vi "仪器电源管理.vi"() -> ()   [LabVIEW 2016, in "环境动力监测库.lvlib" / "电源管理库.lvlib"]
uses:
  <vilib>/Utility/miscctls.llb/LVPointTypeDef.ctl
panel:
  out "R115":i16 caption="灯带关闭时间"
  out "R114":i16 caption="灯带开启时间"
  in  "视频监控":bool
  in  "照明":bool
  in  "前门灯带":bool
  in  "侧边灯带":bool
  in  "电源控制":T1
  in  "副屏看门狗启用":u16(ring) caption="副屏看门狗启用：" items=["关闭", "打开"]
  in  "副屏看门狗设置":u16 caption="副屏看门狗设置："
  out "副屏看门狗计时":u16 caption="副屏看门狗计时："
  in  "主屏看门狗启用":u16(ring) caption="主屏看门狗启用：" items=["关闭", "打开"]
  in  "主屏看门狗设置":u16 caption="主屏看门狗设置："
  out "主屏看门狗计时":u16 caption="主屏看门狗计时："
  # "仪器电源管理"
  # "s"
  # "s"
  # "s"
  # "s"
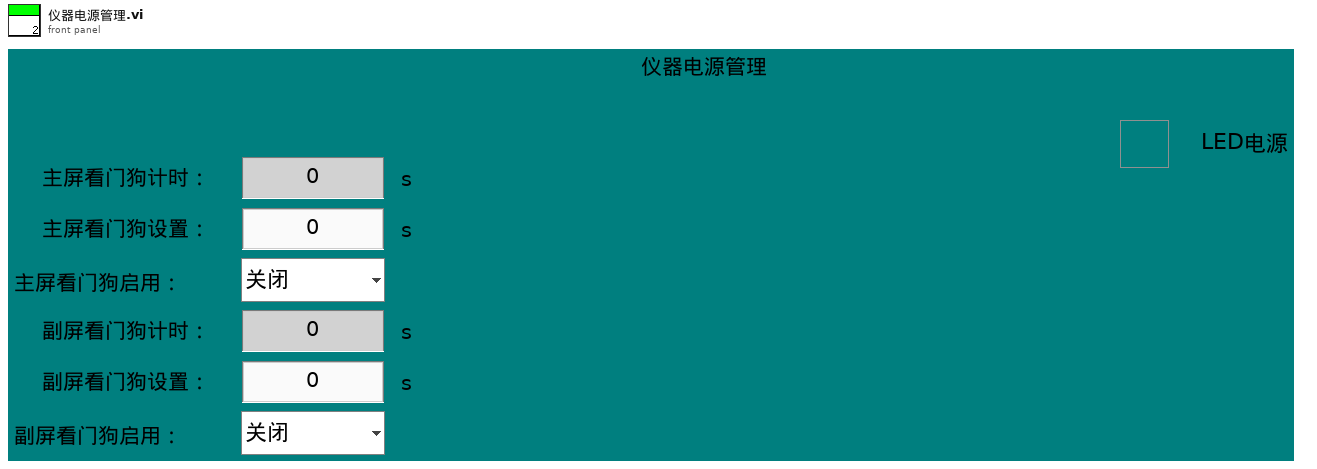
[diagram p1: front panel]
types:
  T1 = cluster{"氨氮电源":bool, "总磷电源":bool, "总氮电源":bool, "多参数电源":bool, "CODMn电源":bool, "CODCr电源":bool, "LED电源":bool}
  T2 = typedef "LVPointTypeDef.ctl" = cluster{"Horizontal":i16, "Vertical":i16}
  T3 = cluster{"采配水启用":bool, "CODMn启用":bool, "CODcr启用":bool, "氨氮启用":bool, "总磷启用":bool, "质控单元启用":bool, "流量计启用":bool, "电源管理启用":bool, "其他启用":bool, "多参数启用":bool, "超标留样启用":bool, "总氮启用":bool, "运行模式":enum16{"维护模式", "常规模式", "应急模式", "质控模式"}}
  T4 = cluster{"状态":cluster{"R0":i16, "R1":i16, "R2":i16, "R3":i16, "R4":i16, "R5":i16, "R6":i16, "R7":i16, "R8":i16, "R9":i16, "R10":i16, "R11":i16, "R12":i16, "R13":i16, "R14":i16, "R15":i16, "R16":i16, "R17":i16, "R18":i16, "R19":i16, "R20":i16, "R21":i16, "R22":i16, "R23":i16, "R24":i16, "R25":i16, "R26":i16, "R27":i16, "R28":i16, "R29":i16, "R30":i16, "R31":i16, "R32":i16, "R33":i16, "R34":i16, "R35":i16, "R36":i16, "R37":i16, "R38":i16, "R39":i16}, "输入状态":bool[], "输出状态":bool[], "参数设置":cluster{"R100":i16, "R101":i16, "R102":i16, "R103":i16, "R104":i16, "R105":i16, "R106":i16, "R107":i16, "R108":i16, "R109":i16, "R110":i16, "R111":i16, "R112":i16, "R113":i16, "R114":i16, "R115":i16, "R116":i16, "R117":i16, "R118":i16, "R119":i16, "R120":i16, "R121":i16, "R122":i16, "R123":i16}, "转换值":cluster{"AD0":sgl, "AD1":sgl, "AD2":sgl, "AD3":sgl, "AD4":sgl, "AD5":sgl}}
  T5 = cluster{"R100":i16, "R101":i16, "R102":i16, "R103":i16, "R104":i16, "R105":i16, "R106":i16, "R107":i16, "R108":i16, "R109":i16, "R110":i16, "R111":i16, "R112":i16, "R113":i16, "R114":i16, "R115":i16, "R116":i16, "R117":i16, "R118":i16, "R119":i16, "R120":i16, "R121":i16, "R122":i16, "R123":i16}
  T6 = cluster{"R0":i16, "R1":i16, "R2":i16, "R3":i16, "R4":i16, "R5":i16, "R6":i16, "R7":i16, "R8":i16, "R9":i16, "R10":i16, "R11":i16, "R12":i16, "R13":i16, "R14":i16, "R15":i16, "R16":i16, "R17":i16, "R18":i16, "R19":i16, "R20":i16, "R21":i16, "R22":i16, "R23":i16, "R24":i16, "R25":i16, "R26":i16, "R27":i16, "R28":i16, "R29":i16, "R30":i16, "R31":i16, "R32":i16, "R33":i16, "R34":i16, "R35":i16, "R36":i16, "R37":i16, "R38":i16, "R39":i16}
  T7 = cluster{"命令":string, "data":cluster{"starting address":u16, "coil values":bool[]}}
  T8 = cluster{"命令":string, "数据":cluster{"starting address":u16, "holding register values":u16[]}}
  T9 = cluster{"命令":string, "数据":cluster{"starting address":u16, "holding register value":u16}}
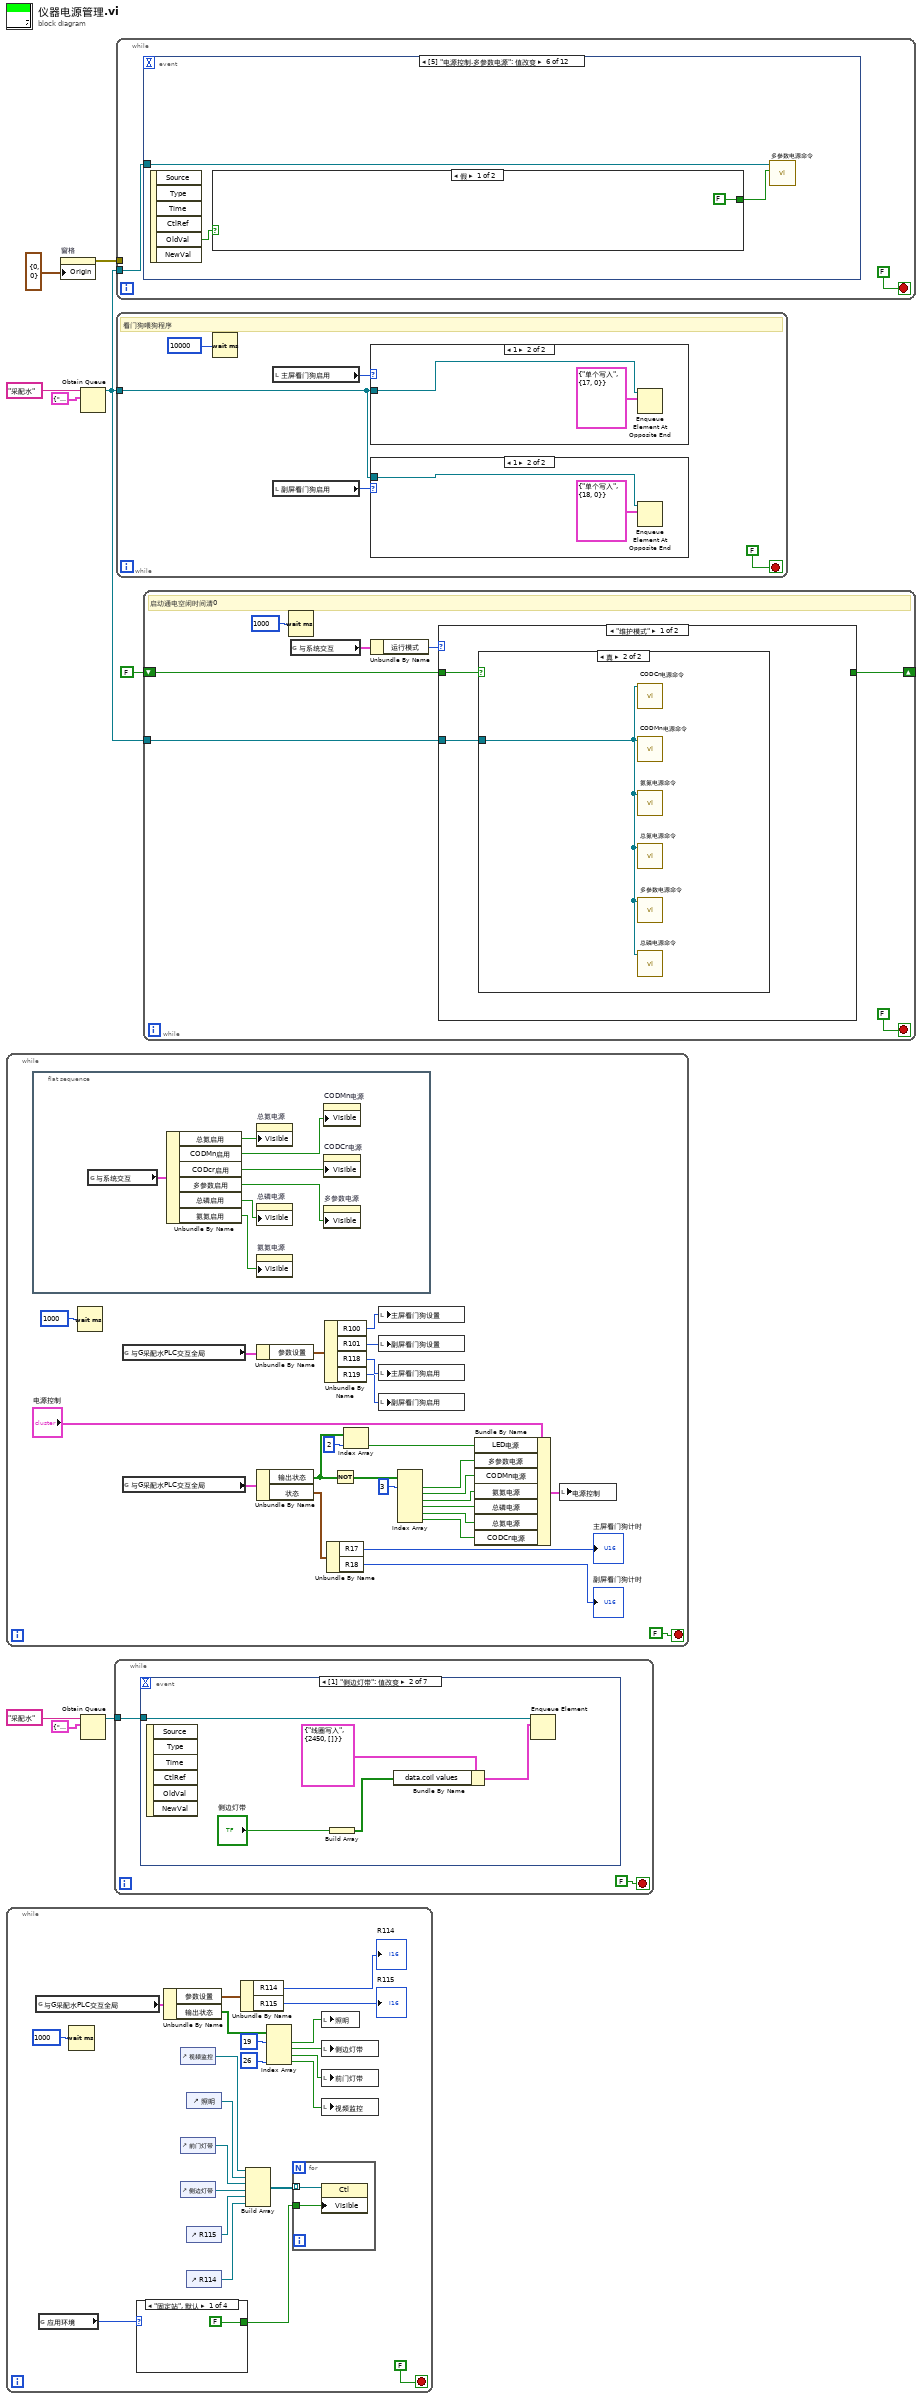
[diagram p0: block diagram]
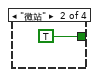
[diagram p2: hidden frame]
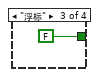
[diagram p3: hidden frame]
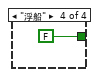
[diagram p4: hidden frame]
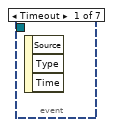
[diagram p5: hidden frame]
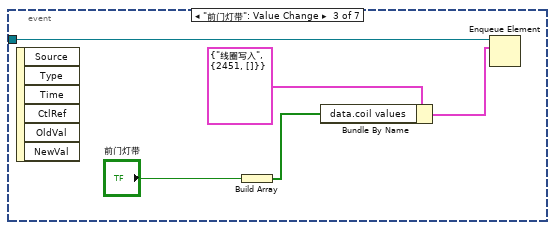
[diagram p6: hidden frame]
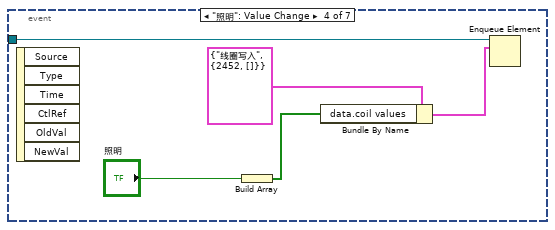
[diagram p7: hidden frame]
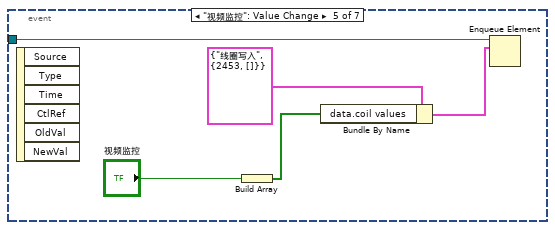
[diagram p8: hidden frame]
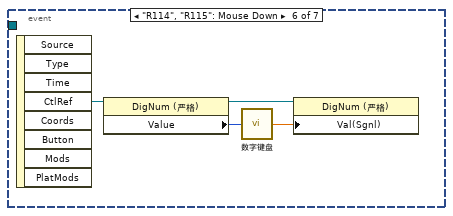
[diagram p9: hidden frame]
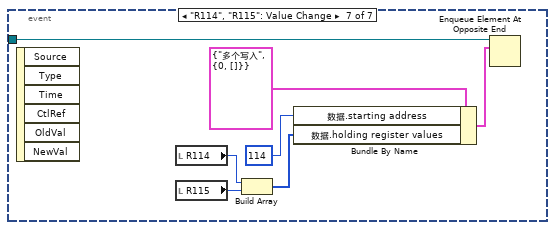
[diagram p10: hidden frame]
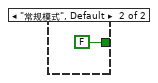
[diagram p14: hidden frame]
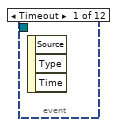
[diagram p15: hidden frame]
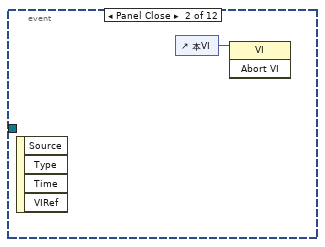
[diagram p16: hidden frame]
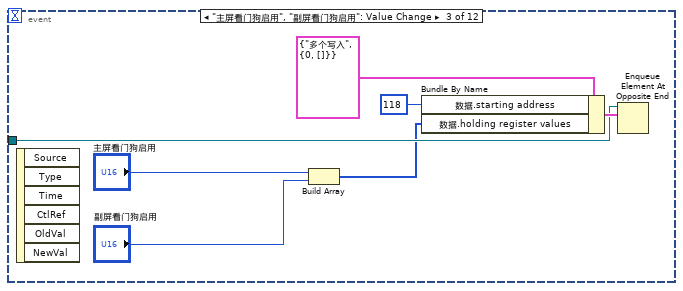
[diagram p17: hidden frame]
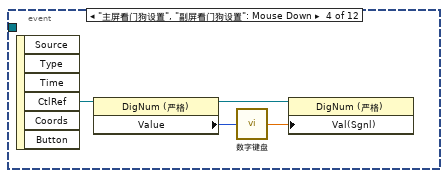
[diagram p18: hidden frame]
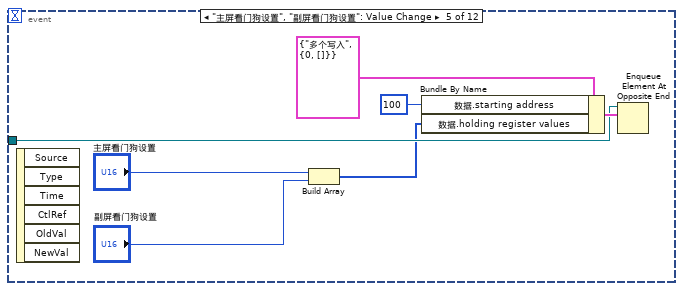
[diagram p19: hidden frame]
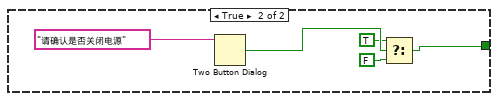
[diagram p20: hidden frame]
diagram:
  n1 = while {
    stop <- FALSE stop-if-true
    n2 = flat-sequence {
      frame #0 {
        n3 = global read "外部交互全局变量.vi" "与系统交互"() -> (w41:T3)
        n4 = Unbundle By Name(w41) -> ("总氮启用"=w40:bool, "CODMn启用"=w39:bool, "CODcr启用"=w35:bool, "多参数启用"=w36:bool, "总磷启用"=w37:bool, "氨氮启用"=w38:bool)
        n5 = property on="总氮电源" class="Bool (严格)"("Visible"=w40) -> ()  [unwired: 2 in, 2 out]
        n6 = property on="总磷电源" class="Bool (严格)"("Visible"=w37) -> ()  [unwired: 2 in, 2 out]
        n7 = property on="氨氮电源" class="Bool (严格)"("Visible"=w38) -> ()  [unwired: 2 in, 2 out]
        n8 = property on="CODMn电源" class="Bool (严格)"("Visible"=w39) -> ()  [unwired: 2 in, 2 out]
        n9 = property on="CODCr电源" class="Bool (严格)"("Visible"=w35) -> ()  [unwired: 2 in, 2 out]
        n10 = property on="多参数电源" class="Bool (严格)"("Visible"=w36) -> ()  [unwired: 2 in, 2 out]
      }
    }
    n11 = Wait (ms)(milliseconds to wait=u32 1000 ("等待时间（毫秒）")) -> ()  [unwired: 1 out]
    n12 = global read "外部交互全局变量.vi" "与G采配水PLC交互全局"() -> (w14:T4)
    n13 = global read "外部交互全局变量.vi" "与G采配水PLC交互全局"() -> (w12:T4)
    n14 = Unbundle By Name(w14) -> ("参数设置"=w13:T5)
    n15 = Unbundle By Name(w12) -> ("输出状态"=w11:bool[], "状态"=w10:T6)
    n16 = Unbundle By Name(w13) -> ("R100"=w29:i16, "R101"=w28:i16, "R118"=w27:i16, "R119"=w26:i16)
    n17 = Unbundle By Name(w10) -> ("R17"=→"主屏看门狗计时":i16, "R18"=→"副屏看门狗计时":i16)
    n18 = Not(x=w11) -> (.not. x?=w32:bool[])
    n19 = Index Array(array=w11, index=2 ("索引")) -> (element=w22:bool)
    n20 = local write "主屏看门狗设置"(w29) -> ()
    n21 = local write "副屏看门狗设置"(w28) -> ()
    n22 = local write "主屏看门狗启用"(w27) -> ()
    n23 = local write "副屏看门狗启用"(w26) -> ()
    n24 = Index Array(array=w32, index #1=3 ("索引")) -> (element #1=w21:bool, element #2=w20:bool, element #3=w19:bool, element #4=w18:bool, element #5=w17:bool, element #6=w16:bool)  [unwired: 5 in]
    n25 = Bundle By Name(cluster="电源控制", "LED电源"=w22, "多参数电源"=w21, "CODMn电源"=w20, "氨氮电源"=w19, "总磷电源"=w18, "总氮电源"=w17, "CODCr电源"=w16) -> (w15:T1)
    n26 = local write "电源控制"(w15) -> ()
  }
  n27 = while {
    stop <- FALSE stop-if-true
    n28 = global read "外部交互全局变量.vi" "与G采配水PLC交互全局"() -> (w44:T4)
    n29 = global read "外部交互全局变量.vi" "应用环境"() -> (w53:enum16{"固定站", "微站", "浮标", "浮船"})
    n30 = Wait (ms)(milliseconds to wait=u32 1000 ("等待时间（毫秒）")) -> ()  [unwired: 1 out]
    n31 = case shown="\"固定站\", 默认" w53 {
      tunnel: [FALSE TRUE FALSE FALSE] -> w45
      frame "固定站", Default {
      }
      frame "微站" {
      }
      frame "浮标" {
      }
      frame "浮船" {
      }
    }
    n32 = Unbundle By Name(w44) -> ("参数设置"=w43:T5, "输出状态"=w42:bool[])
    n33 = control-ref of="视频监控"() -> (w52:refnum<vi>)
    n34 = control-ref of="前门灯带"() -> (w50:refnum<vi>)
    n35 = control-ref of="侧边灯带"() -> (w49:refnum<vi>)
    n36 = control-ref of="照明"() -> (w51:refnum<vi>)
    n37 = control-ref of="R115"() -> (w48:refnum<vi>)
    n38 = control-ref of="R114"() -> (w47:refnum<vi>)
    n39 = Unbundle By Name(w43) -> ("R114"=→"R114":i16, "R115"=→"R115":i16)
    n40 = Build Array(w52, w51, w50, w49, w48, w47) -> (w46:refnum<vi>[])
    n41 = Index Array(array=w42, index #1=19 ("索引"), index #4=26 ("索引")) -> (element #1=w58:bool, element #2=w57:bool, element #3=w59:bool, element #4=w56:bool)  [unwired: 2 in]
    n42 = for {
      tunnel: w46 -> [w65] mode=indexing
      tunnel: w45 -> [w64]
      n43 = property class="Ctl"(reference=w65, "Visible"=w64) -> ()  [unwired: 1 in, 2 out]
    }
    n44 = local write "照明"(w58) -> ()
    n45 = local write "侧边灯带"(w57) -> ()
    n46 = local write "前门灯带"(w59) -> ()
    n47 = local write "视频监控"(w56) -> ()
  }
  n48 = property on="窗格" class="Pane"("Origin"=T2 {"Horizontal"=0, "Vertical"=0} ("原点")) -> (error out=w6:errorcluster)  [unwired: 2 in, 1 out]
  n49 = Obtain Queue(name (unnamed)="采配水" ("名称（未命名）"), element data type=cluster{"命令":string, "数据":variant} {"命令"="", "数据"=variant}) -> (queue out=w4:refnum<queue>)  [unwired: 3 in, 2 out]
  n50 = Obtain Queue(name (unnamed)="采配水" ("名称（未命名）"), element data type=cluster{"命令":string, "数据":variant} {"命令"="", "数据"=variant}) -> (queue out=w1:refnum<queue>)  [unwired: 3 in, 2 out]
  n51 = while {
    tunnel: w1 -> [w70]
    stop <- FALSE stop-if-true
    n52 = event shown="[1] \"侧边灯带\": 值改变" {
      selector: _ -> [_ _ _ _ _ _ _]
      dyn-events: _ -> [_ _ _ _ _ _ _]
      timeout: _ -> [_ _ _ _ _ _ _]
      tunnel: w70 -> [_ w73 w79 w84 w89 _ w96]
      event Timeout {
        n53 = event-data() -> ()  [unwired: 1 in, 3 out]
      }
      event "侧边灯带": Value Change {
        n54 = event-data() -> ()  [unwired: 1 in, 6 out]
        n55 = Build Array("侧边灯带") -> (w72:bool[])
        n56 = Bundle By Name(cluster=T7 {"命令"="线圈写入", "data"={"starting address"=2450, "coil values"=[]}} ("元素"), "data.coil values"=w72) -> (w74:T7)
        n57 = Enqueue Element(queue=w73, element=w74) -> ()  [unwired: 2 in, 3 out]
      }
      event "前门灯带": Value Change {
        n58 = event-data() -> ()  [unwired: 1 in, 6 out]
        n59 = Build Array("前门灯带") -> (w78:bool[])
        n60 = Bundle By Name(cluster=T7 {"命令"="线圈写入", "data"={"starting address"=2451, "coil values"=[]}} ("元素"), "data.coil values"=w78) -> (w80:T7)
        n61 = Enqueue Element(queue=w79, element=w80) -> ()  [unwired: 2 in, 3 out]
      }
      event "照明": Value Change {
        n62 = event-data() -> ()  [unwired: 1 in, 6 out]
        n63 = Build Array("照明") -> (w83:bool[])
        n64 = Bundle By Name(cluster=T7 {"命令"="线圈写入", "data"={"starting address"=2452, "coil values"=[]}} ("元素"), "data.coil values"=w83) -> (w85:T7)
        n65 = Enqueue Element(queue=w84, element=w85) -> ()  [unwired: 2 in, 3 out]
      }
      event "视频监控": Value Change {
        n66 = event-data() -> ()  [unwired: 1 in, 6 out]
        n67 = Build Array("视频监控") -> (w88:bool[])
        n68 = Bundle By Name(cluster=T7 {"命令"="线圈写入", "data"={"starting address"=2453, "coil values"=[]}} ("元素"), "data.coil values"=w88) -> (w90:T7)
        n69 = Enqueue Element(queue=w89, element=w90) -> ()  [unwired: 2 in, 3 out]
      }
      event "R114", "R115": Mouse Down {
        n70 = event-data() -> ("CtlRef"=w95:refnum<vi>)  [unwired: 1 in, 7 out]
        n71 = property class="DigNum (严格)"(reference=w95) -> (reference out=w94:refnum<vi>, "Value"=w93:i16)  [unwired: 1 in, 1 out]
        n72 = call "数字键盘.vi"("OldNumber"=w93) -> ("NewNumber"=w92:sgl)
        n73 = property class="DigNum (严格)"(reference=w94, "Val(Sgnl)"=w92) -> ()  [unwired: 1 in, 2 out]
      }
      event "R114", "R115": Value Change {
        n74 = event-data() -> ()  [unwired: 1 in, 6 out]
        n75 = local read "R114"() -> (w101:i16)
        n76 = local read "R115"() -> (w102:i16)
        n77 = Build Array(w101, w102) -> (w97:i16[])
        n78 = Bundle By Name(cluster=T8 {"命令"="多个写入", "数据"={"starting address"=0, "holding register values"=[]}} ("元素"), "数据.starting address"=u16 114, "数据.holding register values"=w97) -> (w98:T8)
        n79 = Enqueue Element At Opposite End(queue=w96, element=w98) -> ()  [unwired: 2 in, 3 out]
      }
    }
  }
  n80 = while {
    tunnel: w4 -> [w104]
    tunnel: w6 -> [_]
    stop <- FALSE stop-if-true
    n81 = event shown="[5] \"电源控制.多参数电源\": 值改变" {
      selector: _ -> [_ _ _ _ _ _ _ _ _ _ _ _]
      dyn-events: _ -> [_ _ _ _ _ _ _ _ _ _ _ _]
      timeout: _ -> [_ _ _ _ _ _ _ _ _ _ _ _]
      tunnel: w104 -> [_ _ w109 _ w120 w126 w134 w144 w153 w162 w171 w180]
      event Timeout {
        n82 = event-data() -> ()  [unwired: 1 in, 3 out]
      }
      event Panel Close {
        n83 = event-data() -> ()  [unwired: 1 in, 4 out]
        n84 = control-ref of="本VI"() -> (w105:refnum<vi>)
        n85 = invoke class="VI" method="Abort VI"(reference=w105) -> ()  [unwired: 2 in, 3 out]
      }
      event "主屏看门狗启用", "副屏看门狗启用": Value Change {
        n86 = event-data() -> ()  [unwired: 1 in, 6 out]
        n87 = Build Array("主屏看门狗启用", "副屏看门狗启用") -> (w106:u16[])
        n88 = Bundle By Name(cluster=T8 {"命令"="多个写入", "数据"={"starting address"=0, "holding register values"=[]}} ("元素"), "数据.starting address"=u16 118, "数据.holding register values"=w106) -> (w110:T8)
        n89 = Enqueue Element At Opposite End(queue=w109, element=w110) -> ()  [unwired: 2 in, 3 out]
      }
      event "主屏看门狗设置", "副屏看门狗设置": Mouse Down {
        n90 = event-data() -> ("CtlRef"=w113:refnum<vi>)  [unwired: 1 in, 5 out]
        n91 = property class="DigNum (严格)"(reference=w113) -> (reference out=w115:refnum<vi>, "Value"=w116:u16)  [unwired: 1 in, 1 out]
        n92 = call "数字键盘.vi"("OldNumber"=w116) -> ("NewNumber"=w114:sgl)
        n93 = property class="DigNum (严格)"(reference=w115, "Val(Sgnl)"=w114) -> ()  [unwired: 1 in, 2 out]
      }
      event "主屏看门狗设置", "副屏看门狗设置": Value Change {
        n94 = event-data() -> ()  [unwired: 1 in, 6 out]
        n95 = Build Array("主屏看门狗设置", "副屏看门狗设置") -> (w117:u16[])
        n96 = Bundle By Name(cluster=T8 {"命令"="多个写入", "数据"={"starting address"=0, "holding register values"=[]}} ("元素"), "数据.starting address"=u16 100, "数据.holding register values"=w117) -> (w121:T8)
        n97 = Enqueue Element At Opposite End(queue=w120, element=w121) -> ()  [unwired: 2 in, 3 out]
      }
      event "电源控制.多参数电源": Value Change {
        n98 = event-data() -> ("OldVal"=w125:bool)  [unwired: 1 in, 5 out]
        n99 = case shown="假" w125 {
          tunnel: [FALSE ("T button?") w128] -> w124
          frame False {
          }
          frame True {
            n100 = Two Button Dialog(message="请确认是否关闭电源" ("消息")) -> (T button?=w131:bool)  [unwired: 2 in]
            n101 = Select(t=TRUE, s=w131, f=FALSE ("T button?")) -> (s? t:f=w128:bool)
          }
        }
        n102 = call "多参数电源命令.vi"("通电/断电"=w124, "队列"=w126) -> ()  [unwired: 9 in, 1 out]
      }
      event "电源控制.LED电源": Value Change {
        n103 = event-data() -> ("OldVal"=w135:bool)  [unwired: 1 in, 5 out]
        n104 = case shown="假" w135 {
          tunnel: [TRUE ("T button?") w137] -> w133
          frame False {
          }
          frame True {
            n105 = Two Button Dialog(message="请确认是否关闭电源" ("消息")) -> (T button?=w140:bool)  [unwired: 2 in]
            n106 = Select(t=FALSE, s=w140, f=TRUE ("T button?")) -> (s? t:f=w137:bool)
          }
        }
        n107 = call "LED电源命令.vi"("通电/断电"=w133, "队列"=w134) -> ()  [unwired: 9 in, 1 out]
      }
      event "电源控制.CODMn电源": Value Change {
        n108 = event-data() -> ("OldVal"=w143:bool)  [unwired: 1 in, 5 out]
        n109 = case shown="假" w143 {
          tunnel: [FALSE ("T button?") w146] -> w142
          frame False {
          }
          frame True {
            n110 = Two Button Dialog(message="请确认是否关闭电源" ("消息")) -> (T button?=w149:bool)  [unwired: 2 in]
            n111 = Select(t=TRUE, s=w149, f=FALSE ("T button?")) -> (s? t:f=w146:bool)
          }
        }
        n112 = call "CODMn电源命令.vi"("通电/断电"=w142, "队列"=w144) -> ()  [unwired: 9 in, 1 out]
      }
      event "电源控制.氨氮电源": Value Change {
        n113 = event-data() -> ("OldVal"=w152:bool)  [unwired: 1 in, 5 out]
        n114 = case shown="假" w152 {
          tunnel: [FALSE ("T button?") w155] -> w151
          frame False {
          }
          frame True {
            n115 = Two Button Dialog(message="请确认是否关闭电源" ("消息")) -> (T button?=w158:bool)  [unwired: 2 in]
            n116 = Select(t=TRUE, s=w158, f=FALSE ("T button?")) -> (s? t:f=w155:bool)
          }
        }
        n117 = call "氨氮电源命令.vi"("通电/断电"=w151, "队列"=w153) -> ()  [unwired: 9 in, 1 out]
      }
      event "电源控制.总磷电源": Value Change {
        n118 = event-data() -> ("OldVal"=w161:bool)  [unwired: 1 in, 5 out]
        n119 = case shown="假" w161 {
          tunnel: [FALSE ("T button?") w164] -> w160
          frame False {
          }
          frame True {
            n120 = Two Button Dialog(message="请确认是否关闭电源" ("消息")) -> (T button?=w167:bool)  [unwired: 2 in]
            n121 = Select(t=TRUE, s=w167, f=FALSE ("T button?")) -> (s? t:f=w164:bool)
          }
        }
        n122 = call "总磷电源命令.vi"("通电/断电"=w160, "队列"=w162) -> ()  [unwired: 9 in, 1 out]
      }
      event "电源控制.CODCr电源": Value Change {
        n123 = event-data() -> ("OldVal"=w170:bool)  [unwired: 1 in, 5 out]
        n124 = case shown="假" w170 {
          tunnel: [FALSE ("T button?") w173] -> w169
          frame False {
          }
          frame True {
            n125 = Two Button Dialog(message="请确认是否关闭电源" ("消息")) -> (T button?=w176:bool)  [unwired: 2 in]
            n126 = Select(t=TRUE, s=w176, f=FALSE ("T button?")) -> (s? t:f=w173:bool)
          }
        }
        n127 = call "CODCr电源命令.vi"("通电/断电"=w169, "队列"=w171) -> ()  [unwired: 9 in, 1 out]
      }
      event "电源控制.总氮电源": Value Change {
        n128 = event-data() -> ("OldVal"=w178:bool)  [unwired: 1 in, 5 out]
        n129 = case shown="假" w178 {
          tunnel: [FALSE ("T button?") w182] -> w179
          frame False {
          }
          frame True {
            n130 = Two Button Dialog(message="请确认是否关闭电源" ("消息")) -> (T button?=w185:bool)  [unwired: 2 in]
            n131 = Select(t=TRUE, s=w185, f=FALSE ("T button?")) -> (s? t:f=w182:bool)
          }
        }
        n132 = call "总氮电源命令.vi"("通电/断电"=w179, "队列"=w180) -> ()  [unwired: 9 in, 1 out]
      }
    }
  }
  n133 = while {
    tunnel: w4 -> [w191]
    stop <- FALSE stop-if-true
    # "看门狗喂狗程序"
    n134 = Wait (ms)(milliseconds to wait=u32 10000 ("等待时间（毫秒）")) -> ()  [unwired: 1 out]
    n135 = local read "主屏看门狗启用"() -> (w190:u16)
    n136 = local read "副屏看门狗启用"() -> (w189:u16)
    n137 = case shown="1" w190 {
      tunnel: w191 -> [_ w194]
      frame 0, Default {
      }
      frame 1 {
        n138 = Enqueue Element At Opposite End(queue=w194, element=T9 {"命令"="单个写入", "数据"={"starting address"=17, "holding register value"=0}} ("元素")) -> ()  [unwired: 2 in, 3 out]
      }
    }
    n139 = case shown="1" w189 {
      tunnel: w191 -> [_ w192]
      frame 0, Default {
      }
      frame 1 {
        n140 = Enqueue Element At Opposite End(queue=w192, element=T9 {"命令"="单个写入", "数据"={"starting address"=18, "holding register value"=0}} ("元素")) -> ()  [unwired: 2 in, 3 out]
      }
    }
  }
  n141 = while {
    tunnel: w4 -> [w200]
    shift-right: [w198] -> _
    shift-left: FALSE -> [w199]
    stop <- FALSE stop-if-true
    # "启动通电空闲时间清0"
    n142 = Wait (ms)(milliseconds to wait=u32 1000 ("等待时间（毫秒）")) -> ()  [unwired: 1 out]
    n143 = global read "外部交互全局变量.vi" "与系统交互"() -> (w197:T3)
    n144 = Unbundle By Name(w197) -> ("运行模式"=w196:enum16{"维护模式", "常规模式", "应急模式", "质控模式"})
    n145 = case shown="\"维护模式\"" w196 {
      tunnel: w200 -> [w204 _]
      tunnel: w199 -> [w203 _]
      tunnel: [_ FALSE] -> w198
      frame "维护模式" {
        n146 = case shown="真" w203 {
          tunnel: w204 -> [_ w205]
          frame False {
          }
          frame True {
            n147 = call "CODCr电源命令.vi"("队列"=w205) -> ()  [unwired: 10 in, 1 out]
            n148 = call "CODMn电源命令.vi"("队列"=w205) -> ()  [unwired: 10 in, 1 out]
            n149 = call "氨氮电源命令.vi"("队列"=w205) -> ()  [unwired: 10 in, 1 out]
            n150 = call "总氮电源命令.vi"("队列"=w205) -> ()  [unwired: 10 in, 1 out]
            n151 = call "多参数电源命令.vi"("队列"=w205) -> ()  [unwired: 10 in, 1 out]
            n152 = call "总磷电源命令.vi"("队列"=w205) -> ()  [unwired: 10 in, 1 out]
          }
        }
      }
      frame "常规模式", Default {
      }
    }
  }
